vi "PDF Protokoll EPA1065_ARN.vi"(7 "error in (no error)":errorcluster caption="Fehler (Eingang, kein Fehler)") -> (0 "error out":errorcluster caption="Fehler (Ausgang)")   [LabVIEW 2020]
uses:
  <vilib>/Utility/miscctls.llb/LVPrintingMarginsTypeDef.ctl
  Allgemein/allgemeine Sub-VIs.lvlib
  <vilib>/Utility/miscctls.llb/LVRowAndColumnTypeDef.ctl
  Aktion FGV Protokoll.ctl
panel:
  out "Graph1":waveform(dbl)(graph)
  out "Tabelle 3":string[][](table)
  out "Tabelle 2":string[][](table)
  out "Tabelle":string[][](table)
  # "ARN - Test  EPA § 1065.305"
  # "IAG-Prüfstandstechnik GmbH    l Industriestraße 322    l   2722Weikersdorf     www.iag-ng.at"
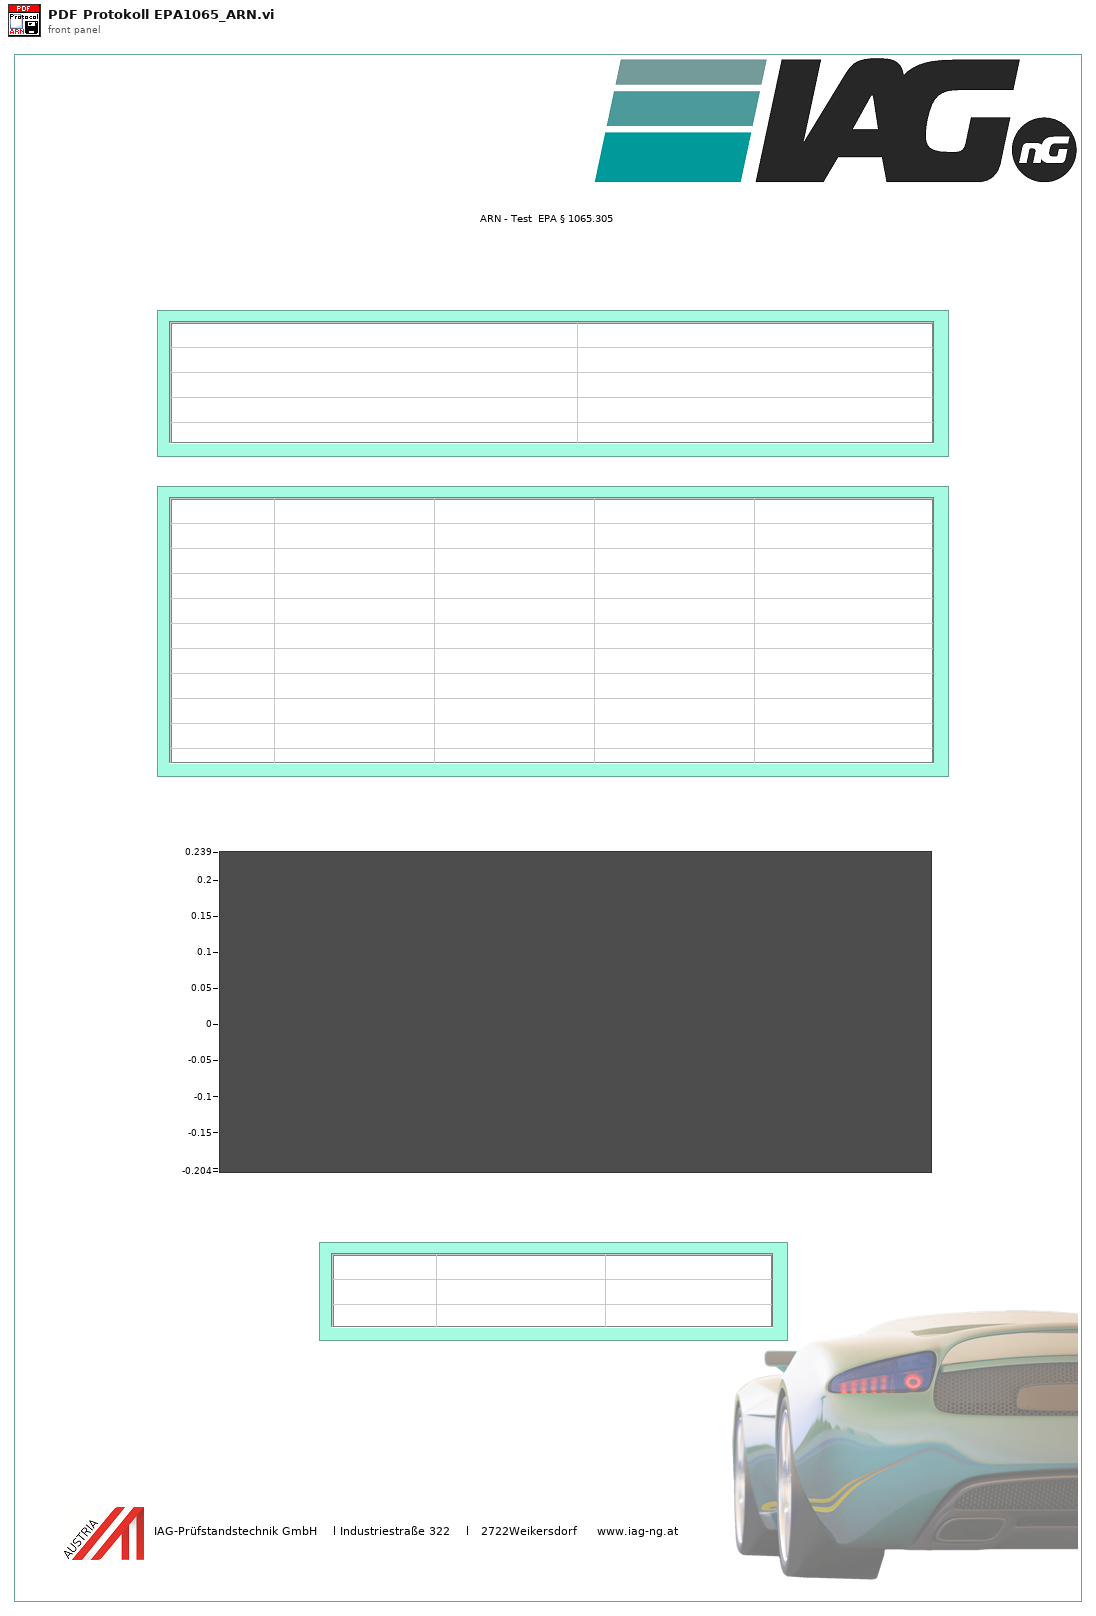
[diagram p1: front panel]
types:
  T1 = typedef "EPA 1065.lvlib/ARN Test 1065-305.lvlib/Aktion FGV Protokoll.ctl" = enum16{"lesen", "schreiben", "Graph"}
  T2 = typedef "LVRowAndColumnTypeDef.ctl" = cluster{"Row":i32, "Column":i32}
  T3 = enum32{"Portrait", "Landscape", "Rotated Portrait", "Rotated Landscape"}
  T4 = typedef "LVPrintingMarginsTypeDef.ctl" = cluster{"Top":sgl, "Left":sgl, "Bottom":sgl, "Right":sgl, "Measurement System":enum8{"Inches", "cm"}}
  T5 = typedef "EPA 1065.lvlib/ARN Test 1065-305.lvlib/Cluster PDF.ctl" = cluster{"TAB 1":T6[][], "TAB 2":string[][], "TAB 3":string[][], "Error":bool[]}
  T6 = typedef "String - Ausgabefeld.ctl" = string
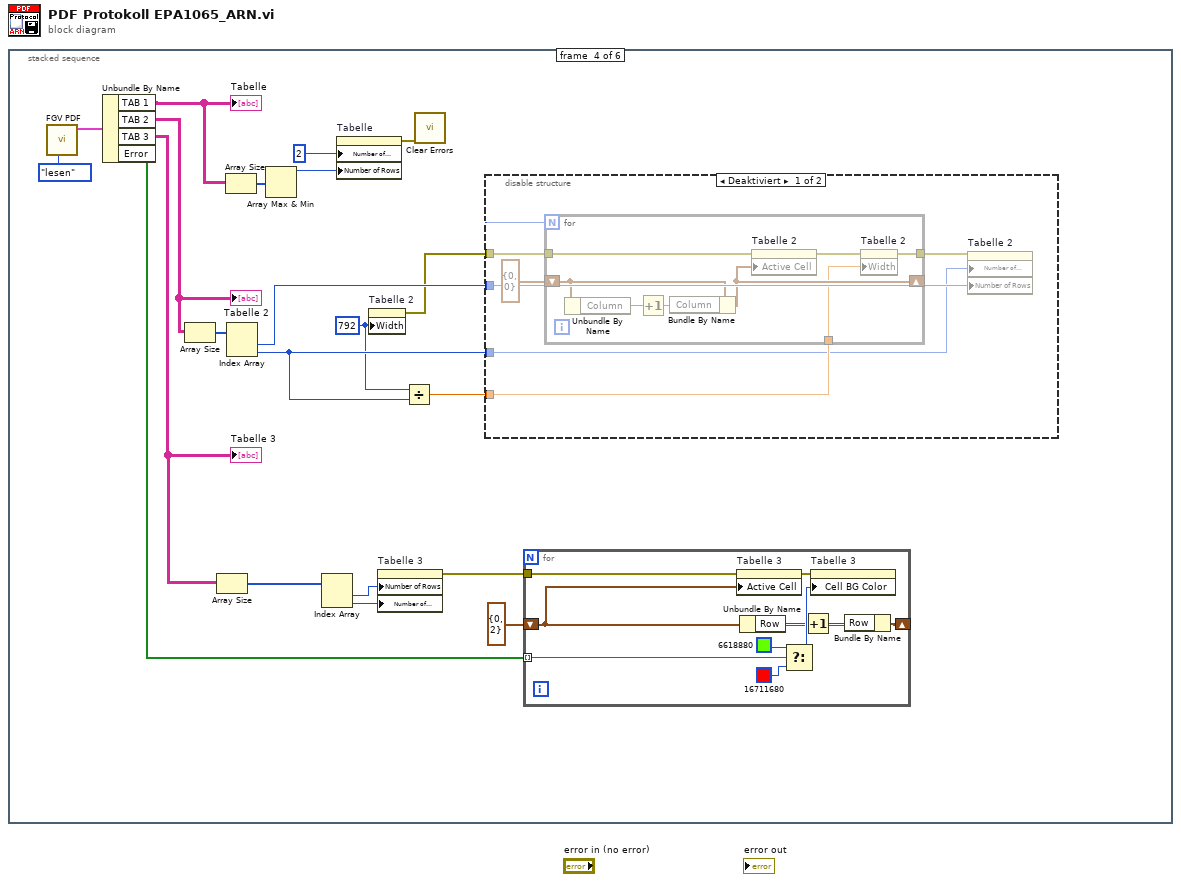
[diagram p0: block diagram]
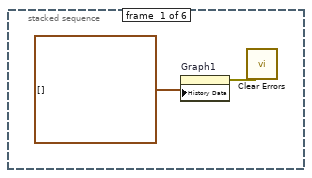
[diagram p2: hidden frame]
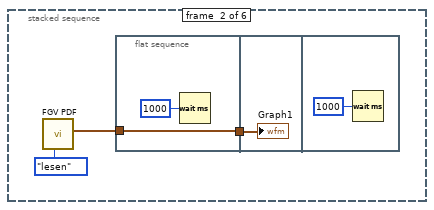
[diagram p3: hidden frame]
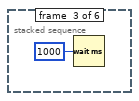
[diagram p4: hidden frame]
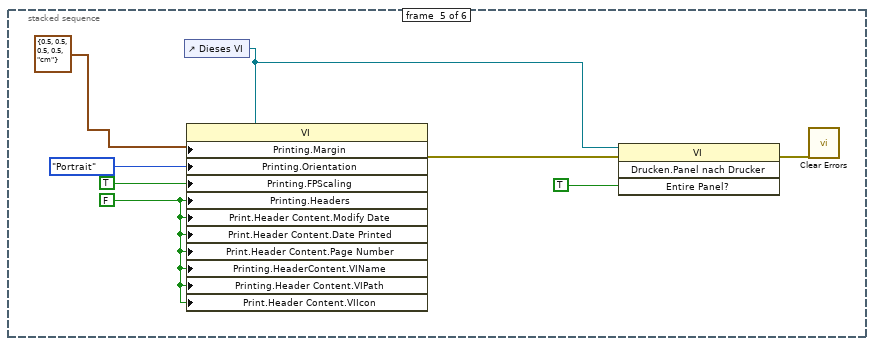
[diagram p6: hidden frame]
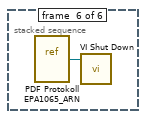
[diagram p7: hidden frame]
diagram:
  n1 = stacked-sequence {
    frame #0 {
      n2 = property on="Graph1" class="SVDiagr (strikt)"("History Data"=waveform(dbl)[] [] ("Historiendaten")) -> (error out=w1:errorcluster)  [unwired: 2 in, 1 out]
      n3 = call <vilib>:"Clear Errors.vi"("error in (no error)"=w1) -> ()  [unwired: 5 in, 2 out]
    }
    frame #1 {
      n4 = call "FGV PDF.vi"("Aktion"=Aktion_FGV_Protokoll."lesen") -> ("Graph"=w3:waveform(dbl))  [unwired: 9 in, 1 out]
      n5 = flat-sequence {
        tunnel: w3 -> [w7]
        tunnel: [w7] -> w4
        tunnel: w4 -> [w8]
        frame #0 {
          n6 = Wait (ms)(milliseconds to wait=u32 1000 ("ms")) -> ()  [unwired: 1 out]
        }
        frame #1 {
          "Graph1" <- w8
        }
        frame #2 {
          n7 = Wait (ms)(milliseconds to wait=u32 1000 ("ms")) -> ()  [unwired: 1 out]
        }
      }
    }
    frame #2 {
      n8 = Wait (ms)(milliseconds to wait=u32 1000 ("Zu wartende ms")) -> ()  [unwired: 1 out]
    }
    frame #3 {
      w11 = u32 792 ("Größe:Breite")
      n9 = call "FGV PDF.vi"("Aktion"=Aktion_FGV_Protokoll."lesen") -> ("Cluster"=w12:T5)  [unwired: 9 in, 1 out]
      n10 = Unbundle By Name(w12) -> ("TAB 1"=w17:T6[][], "TAB 2"=w16:string[][], "TAB 3"=w15:string[][], "Error"=w14:bool[])
      "Tabelle" <- w17
      "Tabelle 2" <- w16
      "Tabelle 3" <- w15
      n11 = Array Size(array=w16) -> (size(s)=w27:i32[])
      n12 = Array Size(array=w15) -> (size(s)=w22:i32[])
      n13 = Array Size(array=w17) -> (size(s)=w29:i32[])
      n14 = Index Array(array=w27) -> (element #1=w26:i32, element #2=w24:i32)  [unwired: 2 in]
      n15 = Array Max & Min(array=w29) -> (max value=w28:i32)  [unwired: 3 out]
      n16 = Index Array(array=w22) -> (element #1=w20:i32, element #2=w19:i32)  [unwired: 2 in]
      n17 = property on="Tabelle" class="Tbl (strikt)"("Number of Columns"=u32 2 ("Spaltenanzahl"), "Number of Rows"=w28) -> (error out=w30:errorcluster)  [unwired: 2 in, 1 out]
      n18 = property on="Tabelle 2" class="Tbl (strikt)"("Width"=w11) -> (error out=w23:errorcluster)  [unwired: 2 in, 1 out]
      n19 = property on="Tabelle 3" class="Tbl (strikt)"("Number of Rows"=w20, "Number of Columns"=w19) -> (error out=w21:errorcluster)  [unwired: 2 in, 1 out]
      n20 = Divide(x=w11, y=w24) -> (x/y=w25:dbl)
      n21 = call <vilib>:"Clear Errors.vi"("error in (no error)"=w30) -> ()  [unwired: 5 in, 2 out]
      n22 = disable-structure shown="Deaktiviert" {
        disable-tunnel: w26 -> [w37 _]
        disable-tunnel: w25 -> [w36 _]
        disable-tunnel: w24 -> [w34 _]
        disable-tunnel: w23 -> [w32 _]
        frame Disabled {
          n23 = for {
            N: w34 -> [_]
            tunnel: w36 -> [w39]
            tunnel: [w42] -> w33
            tunnel: w32 -> [w41]
            shift-right: [w40] -> _
            shift-left: T2 {"Row"=0, "Column"=0} ("Aktive Zelle:Aktive Zelle") -> [w38]
            n24 = Unbundle By Name(w38) -> ("Column"=w44:i32)
            n25 = Increment(x=w44) -> (x+1=w43:i32)
            n26 = Bundle By Name(cluster=w38, "Column"=w43) -> (w40:T2)
            n27 = property on="Tabelle 2" class="Tbl (strikt)"(error in=w41, "Active Cell"=w40) -> (error out=w45:errorcluster)  [unwired: 1 in, 1 out]
            n28 = property on="Tabelle 2" class="Tbl (strikt)"(error in=w45, "Width"=w39) -> (error out=w42:errorcluster)  [unwired: 1 in, 1 out]
          }
          n29 = property on="Tabelle 2" class="Tbl (strikt)"(error in=w33, "Number of Columns"=w34, "Number of Rows"=w37) -> ()  [unwired: 1 in, 2 out]
        }
        frame Enabled {
        }
      }
      n30 = for {
        tunnel: w21 -> [w55]
        tunnel: w14 -> [w53] mode=indexing
        shift-right: [w46] -> _
        shift-left: T2 {"Row"=0, "Column"=2} ("Aktive Zelle:Aktive Zelle") -> [w47]
        n31 = property on="Tabelle 3" class="Tbl (strikt)"(error in=w55, "Active Cell"=w47) -> (error out=w54:errorcluster)  [unwired: 1 in, 1 out]
        n32 = Unbundle By Name(w47) -> ("Row"=w48:i32)
        n33 = Select(t=u32 6618880, s=w53, f=u32 16711680) -> (s? t:f=w50:u32)
        n34 = Increment(x=w48) -> (x+1=w49:i32)
        n35 = property on="Tabelle 3" class="Tbl (strikt)"(error in=w54, "Cell BG Color"=w50) -> ()  [unwired: 1 in, 2 out]
        n36 = Bundle By Name(cluster=w47, "Row"=w49) -> (w46:T2)
      }
    }
    frame #4 {
      w59 = FALSE ("Drucken:Kopfzeilen?")
      n37 = control-ref of="Dieses VI"() -> (w56:refnum<vi>)
      n38 = property class="VI"(reference=w56, "Printing.Margin"=T4 {"Top"=0.5, "Left"=0.5, "Bottom"=0.5, "Right"=0.5, "Measurement System"=enum."cm"} ("Drucken:Ränder"), "Printing.Orientation"=T3."Portrait" ("Drucken:Seitenausrichtung"), "Printing.FPScaling"=TRUE ("Drucken:Frontpanel-Skalierung?"), "Printing.Headers"=w59, "Print.Header Content.Modify Date"=w59, "Print.Header Content.Date Printed"=w59, "Print.Header Content.Page Number"=w59, "Printing.HeaderContent.VIName"=w59, "Printing.Header Content.VIPath"=w59, "Print.Header Content.VIIcon"=w59) -> (error out=w63:errorcluster)  [unwired: 1 in, 1 out]
      n39 = invoke class="VI" method="Drucken.Panel nach Drucker"(reference=w56, error in=w63, "Entire Panel?"=TRUE ("Abschnittskopfzeilen?")) -> (error out=w57:errorcluster)  [unwired: 1 in, 3 out]
      n40 = call <vilib>:"Clear Errors.vi"("error in (no error)"=w57) -> ()  [unwired: 5 in, 2 out]
    }
    frame #5 {
      n41 = vi-ref "PDF Protokoll EPA1065_ARN.vi"() -> (w64:refnum<vi>)
      n42 = call "VI Shut Down.vi"("VI Referenz"=w64) -> ()  [unwired: 11 in]
    }
  }
